vi "Cancel Tasks.vi"(8 "error in (no error)":errorcluster, 11 "BuildServer in":refnum<class "BuildServer.lvclass">) -> (0 "error out":errorcluster, 3 "BuildServer out":refnum<class "BuildServer.lvclass">)   [LabVIEW 2017, in "BuildServer.lvlib" / "BuildServer.lvclass"]
uses:
  BuildServer.lvclass
  BuildServer.lvclass/BuildServer.ctl
  Classes/Comm Interface/Comm Interface.lvclass
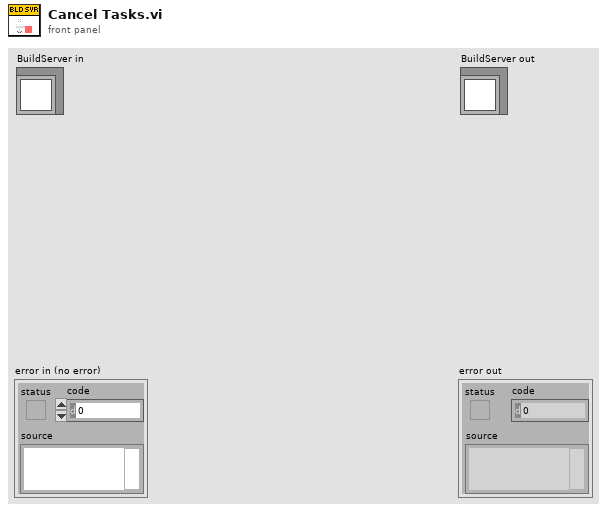
[diagram p1: front panel]
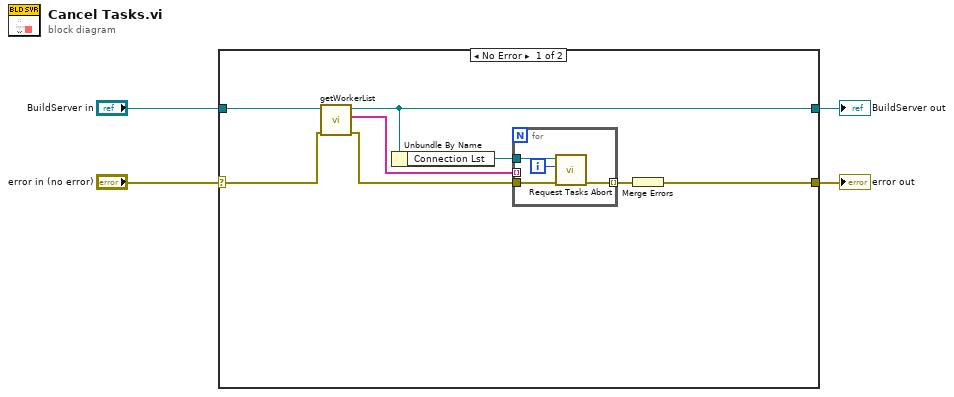
[diagram p0: block diagram]
diagram:
  n1 = case shown="No Error" "error in (no error)" {
    selector: "error in (no error)" -> [w7 w18]
    tunnel: [w5 w18] -> w3
    tunnel: [w11 w17] -> w1
    tunnel: "BuildServer in" -> [w12 w17]
    frame No Error {
      n2 = call "getWorkerList.vi"("error in (no error)"=w7, "BuildServer in"=w12) -> ("error out"=w8:errorcluster, "Worker List"=w10:string[], "BuildServer out"=w11:refnum<class "BuildServer.lvclass">)  [unwired: 7 in]
      n3 = Unbundle By Name(w11) -> ("Connection Lst"=w9:refnum<class "Comm Interface.lvclass">)
      n4 = for {
        tunnel: w10 -> [_] mode=indexing
        tunnel: w9 -> [w16]
        tunnel: w8 -> [w14]
        tunnel: [w13] -> w6 mode=indexing
        i -> [w15]
        n5 = call "Request Tasks Abort.vi"("error in (no error)"=w14, "index"=w15, "Comm Interface in"=w16) -> ("error out"=w13:errorcluster)  [unwired: 7 in, 1 out]
      }
      n6 = Merge Errors(w6) -> (w5:errorcluster)
    }
    frame Error {
    }
  }
  "error out" <- w3
  "BuildServer out" <- w1
